vi "Config_PXDAC4800_2.vi"(0 "NumBoard":u32=1, 5 "Config":T2={"Clock source"=enum."1200 MHz", "Active channel"=enum."Dual channel - Ch1 & Ch2", "Trigger direction"=enum."Positive (Rising edge)", "Trigger mode"=enum."Continuous", "External Trigger enable"=FALSE, "Dac sample size"=enum."14 Bits LSB\n", "Dac sample format"=enum."Unsigned", "ClkDiv1"=1, "ClkDiv2"=1, "Output voltage level - Ch1"=1023, "Output voltage level - Ch2"=1023, "Output voltage level - Ch3"=1023, "Output voltage level - Ch4"=1023} {"Output voltage level - Ch4" min=1 max=1023 step=1 scale=0.0..1023.0; "Output voltage level - Ch3" min=1 max=1023 step=1 scale=0.0..1023.0; "Output voltage level - Ch2" min=1 max=1023 step=1 scale=0.0..1023.0; "Output voltage level - Ch1" min=1 max=1023 step=1 scale=0.0..1023.0}) -> (6 "Handle":u32=215368648, 8 "Serial num":u32=301738, 10 "Status":i32, 15 "Error/output message":string="SUCCESS")   [LabVIEW 2016]
panel:
  out "x+y":dbl=1.9797466172610085
  out "x*y":dbl=0.35000000000000003
  in  "NumBoard 3":u32=1
  in  "NumBoard 2":u32=1
  out "Serial num 3":u32=301738
  out "Handle 4":u32=266145720
  out "Status 4":i32
  out "Error/output message 4":string="SUCCESS"
  in  "Create Waveform":bool=TRUE
  in  "Playback":bool=TRUE
  in  "Configure":bool
  in  "Tab Control":T1(tab)=enum."Create Waveform"
  in  "DAC frequency (MHz)":dbl=1200.0
  in  "Number Of Points(integer multiple of 4096)":i32=30
  in  "Envelope Decay Time (micro s)":dbl=0.1
  in  "Amplitude (Max 1.4 V)":dbl=1.3
  in  "Frequency (MHz)":dbl=220.0
  out "output waveform":waveform(dbl)(graph)={"t0"=timestamp(0 s since 1904-01-01), "dt"=0.0008333333333333334, "Y"=array[122880 elements]}
  out "output waveform 2":waveform(dbl)(graph)={"t0"=timestamp(0 s since 1904-01-01), "dt"=0.0008333333333333334, "Y"=array[122880 elements]}
  in  "Shaped Wave Packet":bool=TRUE
  in  "Duty Cycle":dbl=2.0
  in  "Pulse Center":dbl=4.0
  in  "Square Pulse Amplitude":dbl=1.4 format="%#_13g"
  in  "Pulsed":bool=TRUE
  in  "VISA Refnum in":refnum<visa-resource-name>="USB0::0x0699::0x0353::1650390::INSTR"
  in  "time(us) 2":dbl=1.0
  out "Status 2":i32
  out "Handle 2":u32=266146304
  out "Serial num 2":u32=301738
  in  "dst_offset_bytes":u32
  in  "dst_length_bytes":u32
  in  "src_offset_bytes":u32
  in  "src_length_bytes":u32
  in  "Offset":u32
  in  "Length":u32
  out "Error/output message 3":string="SUCCESS"
  out "Channel":i32=3
  out "Handle 3":u32=264143912
  out "Status 3":i32
  in  "Run":bool=TRUE
  out "Error/output message 2":string="SUCCESS"
  in  "File":path=path "C:/Program Files (x86)/Signatec/PXDAC4800/version5.rd16"
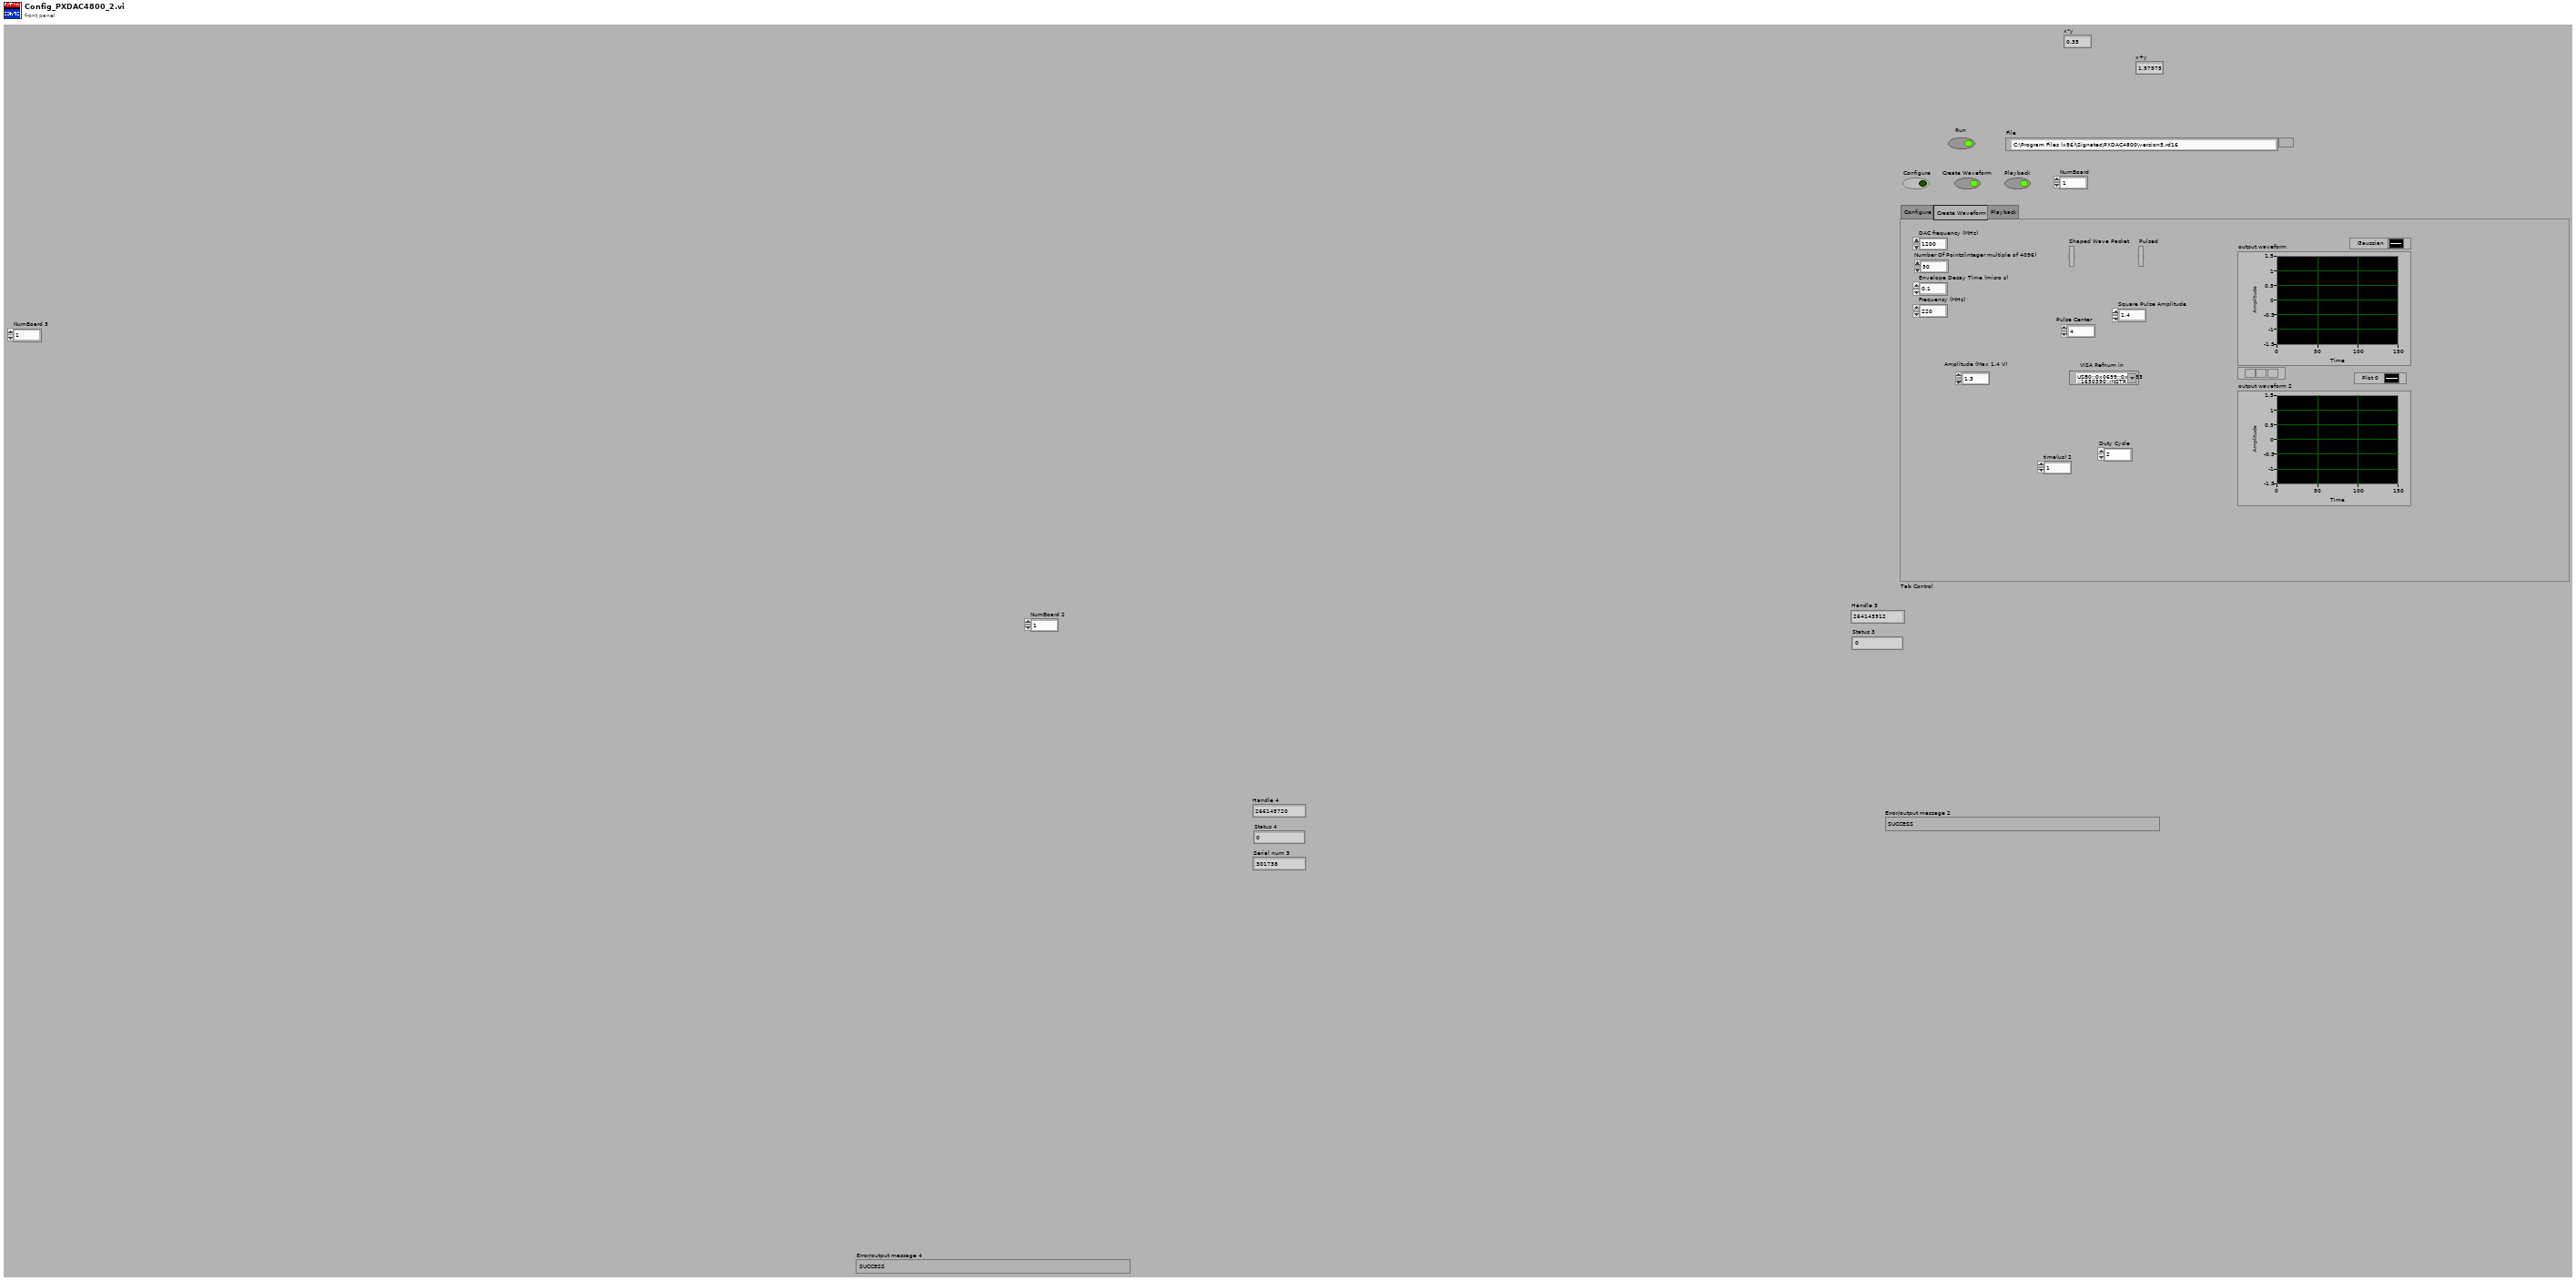
[diagram p1: front panel]
types:
  T1 = enum32{"Configure", "Create Waveform", "Playback"}
  T2 = cluster{"Clock source":enum16{"1200 MHz", "900 MHz", "External"}, "Active channel":enum16{"Dual channel - Ch1 & Ch2", "Single channel - Ch1"}, "Trigger direction":enum16{"Positive (Rising edge)", "Negative (Falling edge)"}, "Trigger mode":enum16{"Per trigger", "Continuous", "Single shot"}, "External Trigger enable":bool, "Dac sample size":enum16{"8 bits", "14 bits MSB", "14 Bits LSB\n"}, "Dac sample format":enum16{"Unsigned", "Signed"}, "ClkDiv1":u32, "ClkDiv2":u32, "Output voltage level - Ch1":u32, "Output voltage level - Ch2":u32, "Output voltage level - Ch3":u32, "Output voltage level - Ch4":u32}
  T3 = enum16{"Connect", "EndRamPlaybackXD48", "Disconnect"}
  T4 = enum16{"Connect", "GetSerialNumber", "SetActiveChannelMaskXD48", "SetPlaybackClockSourceXD48", "SetClockDivider1XD48", "SetClockDivider2XD48", "SetOutputVoltageCh1XD48", "SetOutputVoltageCh2XD48", "SetOutputVoltageCh3XD48", "SetOutputVoltageCh4XD48", "SetDacSampleFormatXD48", "SetDacSampleSizeXD48", "SetExternalTriggerEnableXD48", "SetExternalTriggerDirXD48", "SetTriggerModeXD48", "Disconnect"}
  T5 = enum16{"Dual channel - Ch1 & Ch2", "Single channel - Ch1"}
  T6 = enum16{"Positive (Rising edge)", "Negative (Falling edge)"}
  T7 = enum16{"Per trigger", "Continuous", "Single shot"}
  T8 = enum16{"Connect", "GetSerialNumber", "EndRamPlaybackXD48"}
  T9 = enum16{"Connect", "GetSerialNumber", "LoadFileIntoRam", "BeginRamPlayback", "Trigger", "EndRamPlaybackXD48", "Disconnect"}
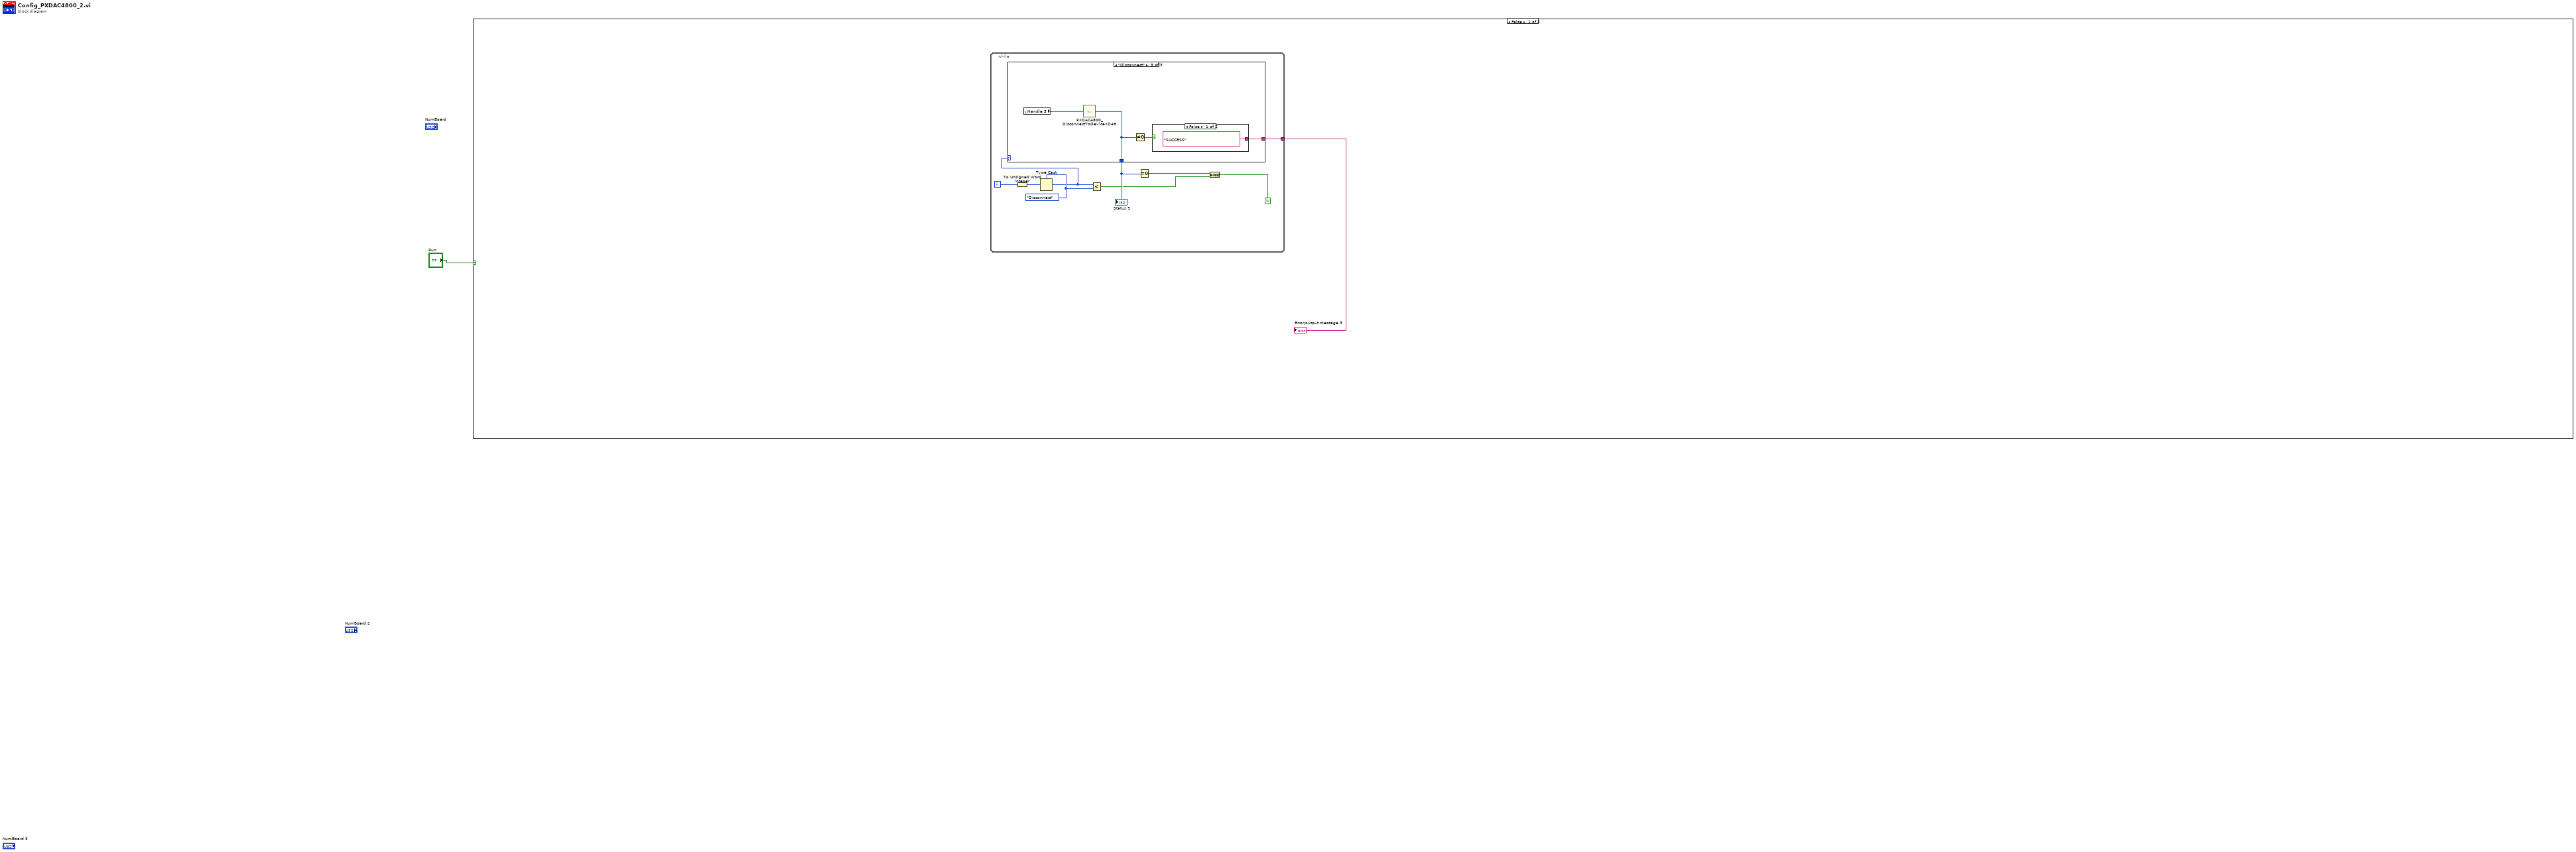
[diagram p0: block diagram]
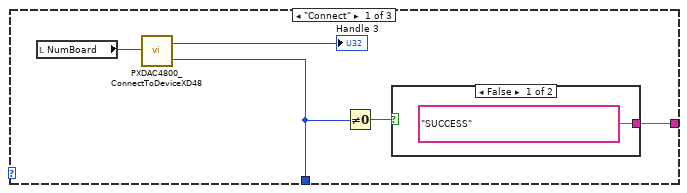
[diagram p2: hidden frame]
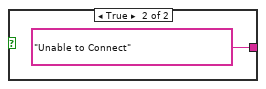
[diagram p3: hidden frame]
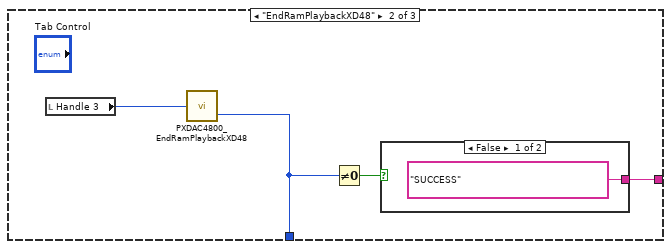
[diagram p4: hidden frame]
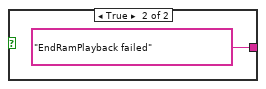
[diagram p5: hidden frame]
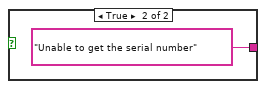
[diagram p6: hidden frame]
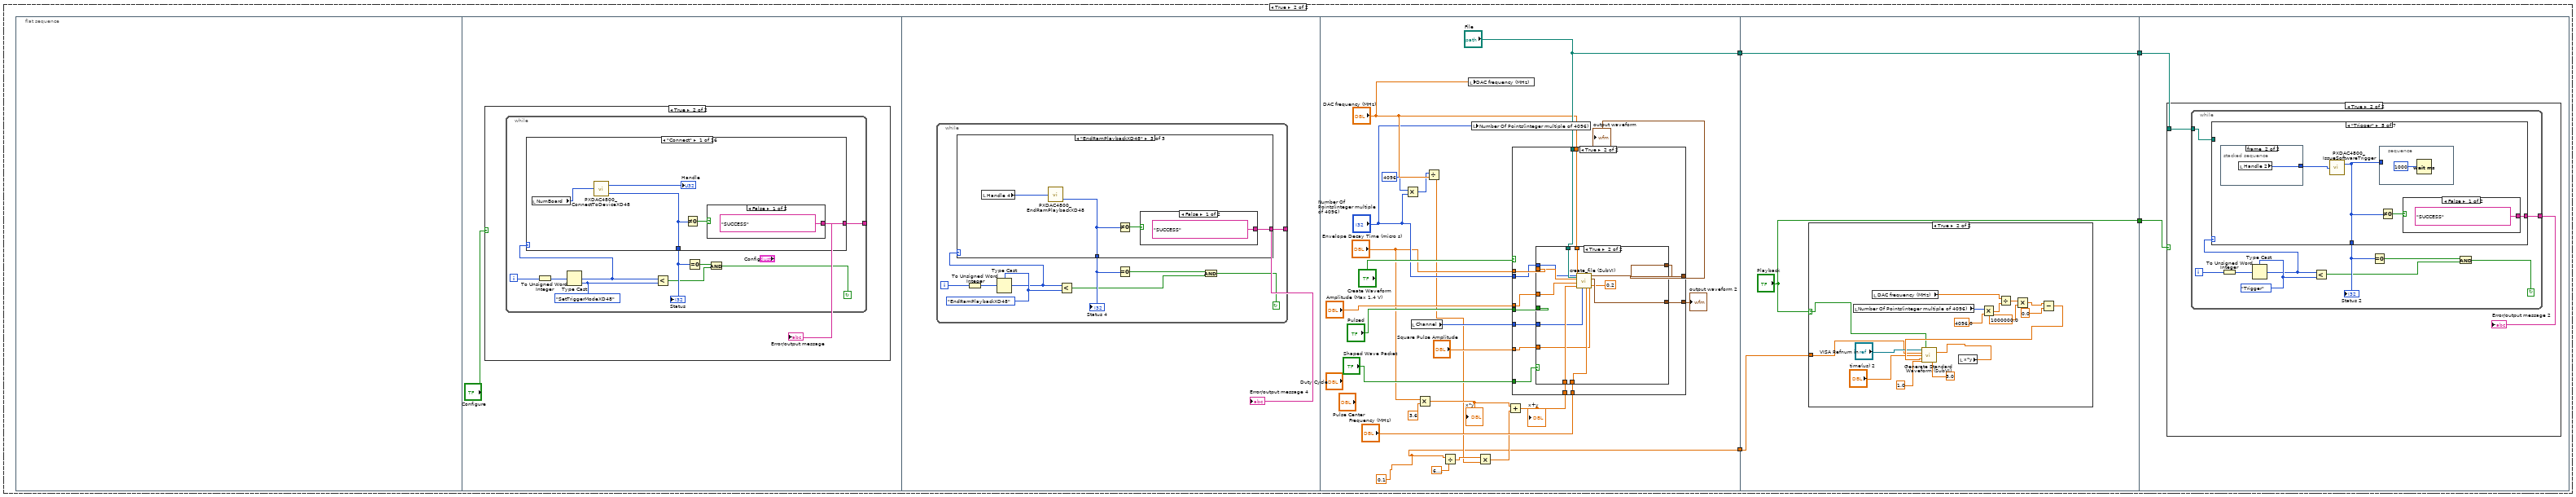
[diagram p7: hidden frame]
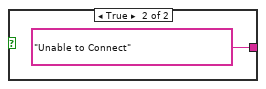
[diagram p9: hidden frame]
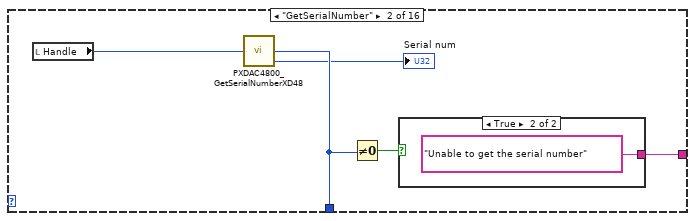
[diagram p10: hidden frame]
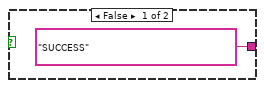
[diagram p11: hidden frame]
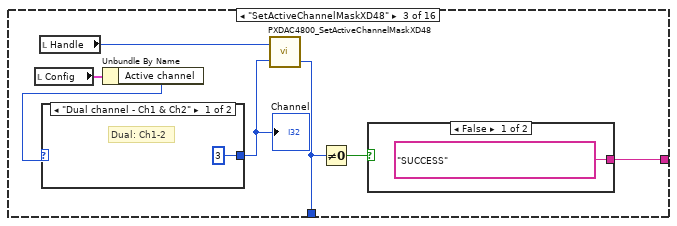
[diagram p12: hidden frame]
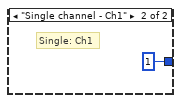
[diagram p13: hidden frame]
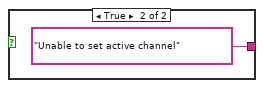
[diagram p14: hidden frame]
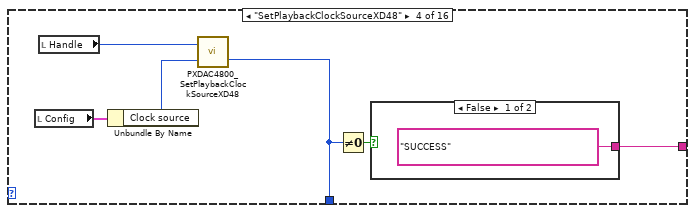
[diagram p15: hidden frame]
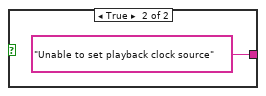
[diagram p16: hidden frame]
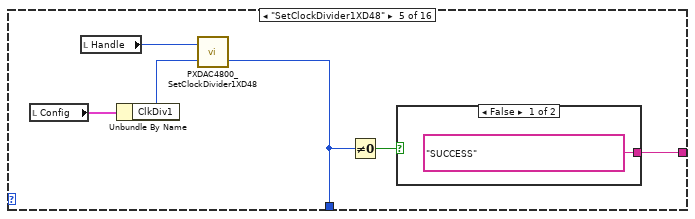
[diagram p17: hidden frame]
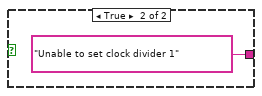
[diagram p18: hidden frame]
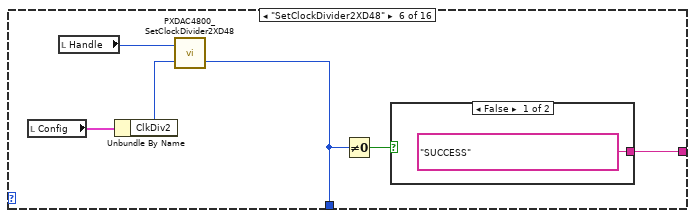
[diagram p19: hidden frame]
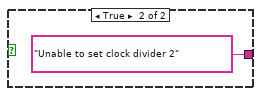
[diagram p20: hidden frame]
diagram:
  n1 = case shown="False" "Run" {
    frame False {
      n2 = while {
        tunnel: [w4] -> w2
        i -> [w11]
        stop <- w5 continue-if-true
        w9 = T3."Disconnect"
        n3 = To Unsigned Word Integer(number=w11) -> (unsigned 16bit integer=w10:u16)
        n4 = Type Cast(type=w9, x=w10) -> (*(type *) &x=w3:T3)
        n5 = case shown="\"Disconnect\"" w3 {
          tunnel: [w13 w19 w25] -> w8
          tunnel: [w15 w21 w28] -> w4
          frame "Connect" {
            n6 = local read "NumBoard"() -> (w12:u32)
            n7 = call "PXDAC4800_ConnectToDeviceXD48.vi"("brdNum"=w12) -> ("Handle Out"=→"Handle 3":i32, "Status"=w13:i32)
            n8 = Not Equal To 0?(x=w13) -> (x != 0?=w16:bool)
            n9 = case shown="False" w16 {
              tunnel: ["SUCCESS" "Unable to Connect"] -> w15
              frame False {
              }
              frame True {
              }
            }
          }
          frame "EndRamPlaybackXD48" {
            n10 = local read "Handle 3"() -> (w20:u32)
            n11 = call "PXDAC4800_EndRamPlaybackXD48.vi"("Handle"=w20) -> ("Status"=w19:i32)  [unwired: 1 out]
            n12 = Not Equal To 0?(x=w19) -> (x != 0?=w22:bool)
            n13 = case shown="False" w22 {
              tunnel: ["SUCCESS" "EndRamPlayback failed"] -> w21
              frame False {
              }
              frame True {
              }
            }
          }
          frame "Disconnect" {
            n14 = local read "Handle 3"() -> (w26:u32)
            n15 = call "PXDAC4800_DisconnectToDeviceXD48.vi"("Handle"=w26) -> ("Status"=w25:i32)
            n16 = Not Equal To 0?(x=w25) -> (x != 0?=w27:bool)
            n17 = case shown="False" w27 {
              tunnel: ["SUCCESS" "Unable to get the serial number"] -> w28
              frame False {
              }
              frame True {
              }
            }
          }
        }
        "Status 3" <- w8
        n18 = Less?(x=w3, y=w9) -> (x < y?=w6:bool)
        n19 = Equal To 0?(x=w8) -> (x = 0?=w7:bool)
        n20 = And(x=w7, y=w6) -> (x .and. y?=w5:bool)
      }
      "Error/output message 3" <- w2
    }
    frame True {
      n21 = flat-sequence {
        tunnel: ["File"] -> w34
        tunnel: [w206] -> w31
        tunnel: w34 -> [w293]
        tunnel: [w293] -> w33
        tunnel: ["Playback"] -> w32
        tunnel: w31 -> [w291]
        tunnel: w33 -> [w311]
        tunnel: w32 -> [w310]
        frame #0 {
        }
        frame #1 {
          n22 = case shown="True" "Configure" {
            frame False {
            }
            frame True {
              n23 = while {
                tunnel: [w37] -> w36
                i -> [w45]
                stop <- w38 continue-if-true
                w42 = T4."SetTriggerModeXD48"
                n24 = To Unsigned Word Integer(number=w45) -> (unsigned 16bit integer=w44:u16)
                n25 = Type Cast(type=w42, x=w44) -> (*(type *) &x=w43:T4)
                n26 = case shown="\"Connect\"" w43 {
                  tunnel: [w47 w55 w64 w74 w81 w89 w97 w105 w113 w121 w129 w137 w145 w156 w164 w170] -> w41
                  tunnel: [w49 w56 w65 w75 w83 w91 w99 w107 w115 w123 w131 w139 w148 w158 w166 w173] -> w37
                  frame "Connect" {
                    n27 = local read "NumBoard"() -> (w46:u32)
                    n28 = call "PXDAC4800_ConnectToDeviceXD48.vi"("brdNum"=w46) -> ("Handle Out"=→"Handle":i32, "Status"=w47:i32)
                    n29 = Not Equal To 0?(x=w47) -> (x != 0?=w50:bool)
                    n30 = case shown="False" w50 {
                      tunnel: ["SUCCESS" "Unable to Connect"] -> w49
                      frame False {
                      }
                      frame True {
                      }
                    }
                  }
                  frame "GetSerialNumber" {
                    (unwired) "Unable to get serial"
                    n31 = local read "Handle"() -> (w53:u32)
                    n32 = call "PXDAC4800_GetSerialNumberXD48.vi"("Handle"=w53) -> ("Status"=w55:i32, "Serial num"=→"Serial num":i32)  [unwired: 1 out]
                    n33 = Not Equal To 0?(x=w55) -> (x != 0?=w57:bool)
                    n34 = case shown="True" w57 {
                      tunnel: ["SUCCESS" "Unable to get the serial number"] -> w56
                      frame False {
                      }
                      frame True {
                      }
                    }
                  }
                  frame "SetActiveChannelMaskXD48" {
                    n35 = local read "Config"() -> (w63:T2)
                    n36 = local read "Handle"() -> (w61:u32)
                    n37 = Unbundle By Name(w63) -> ("Active channel"=w62:T5)
                    n38 = case shown="\"Dual channel - Ch1 & Ch2\"" w62 {
                      tunnel: [3 1] -> w60
                      frame "Dual channel - Ch1 & Ch2" {
                        # "Dual: Ch1-2"
                      }
                      frame "Single channel - Ch1" {
                        # "Single: Ch1"
                      }
                    }
                    "Channel" <- w60
                    n39 = call "PXDAC4800_SetActiveChannelMaskXD48.vi"("Value"=w60, "Handle"=w61) -> ("Status"=w64:i32)  [unwired: 1 out]
                    n40 = Not Equal To 0?(x=w64) -> (x != 0?=w66:bool)
                    n41 = case shown="False" w66 {
                      tunnel: ["SUCCESS" "Unable to set active channel"] -> w65
                      frame False {
                      }
                      frame True {
                      }
                    }
                  }
                  frame "SetPlaybackClockSourceXD48" {
                    n42 = local read "Config"() -> (w72:T2)
                    n43 = local read "Handle"() -> (w73:u32)
                    n44 = Unbundle By Name(w72) -> ("Clock source"=w71:enum16{"1200 MHz", "900 MHz", "External"})
                    n45 = call "PXDAC4800_SetPlaybackClockSourceXD48.vi"("Value"=w71, "Handle"=w73) -> ("Status"=w74:i32)  [unwired: 1 out]
                    n46 = Not Equal To 0?(x=w74) -> (x != 0?=w76:bool)
                    n47 = case shown="False" w76 {
                      tunnel: ["SUCCESS" "Unable to set playback clock source"] -> w75
                      frame False {
                      }
                      frame True {
                      }
                    }
                  }
                  frame "SetClockDivider1XD48" {
                    n48 = local read "Config"() -> (w80:T2)
                    n49 = local read "Handle"() -> (w82:u32)
                    n50 = Unbundle By Name(w80) -> ("ClkDiv1"=w79:u32)
                    n51 = call "PXDAC4800_SetClockDivider1XD48.vi"("Div"=w79, "Handle"=w82) -> ("Status"=w81:i32)  [unwired: 1 out]
                    n52 = Not Equal To 0?(x=w81) -> (x != 0?=w84:bool)
                    n53 = case shown="False" w84 {
                      tunnel: ["SUCCESS" "Unable to set clock divider 1"] -> w83
                      frame False {
                      }
                      frame True {
                      }
                    }
                  }
                  frame "SetClockDivider2XD48" {
                    n54 = local read "Config"() -> (w88:T2)
                    n55 = local read "Handle"() -> (w90:u32)
                    n56 = Unbundle By Name(w88) -> ("ClkDiv2"=w87:u32)
                    n57 = call "PXDAC4800_SetClockDivider2XD48.vi"("Div"=w87, "Handle"=w90) -> ("Status"=w89:i32)  [unwired: 1 out]
                    n58 = Not Equal To 0?(x=w89) -> (x != 0?=w92:bool)
                    n59 = case shown="False" w92 {
                      tunnel: ["SUCCESS" "Unable to set clock divider 2"] -> w91
                      frame False {
                      }
                      frame True {
                      }
                    }
                  }
                  frame "SetOutputVoltageCh1XD48" {
                    n60 = local read "Config"() -> (w96:T2)
                    n61 = local read "Handle"() -> (w98:u32)
                    n62 = Unbundle By Name(w96) -> ("Output voltage level - Ch1"=w95:u32)
                    n63 = call "PXDAC4800_SetOutputVoltageCh1XD48.vi"("Value"=w95, "Handle"=w98) -> ("Status"=w97:i32)  [unwired: 1 out]
                    n64 = Not Equal To 0?(x=w97) -> (x != 0?=w100:bool)
                    n65 = case shown="False" w100 {
                      tunnel: ["SUCCESS" "Unable to set output voltage range ch1"] -> w99
                      frame False {
                      }
                      frame True {
                      }
                    }
                  }
                  frame "SetOutputVoltageCh2XD48" {
                    n66 = local read "Config"() -> (w104:T2)
                    n67 = local read "Handle"() -> (w106:u32)
                    n68 = Unbundle By Name(w104) -> ("Output voltage level - Ch2"=w103:u32)
                    n69 = call "PXDAC4800_SetOutputVoltageCh2XD48.vi"("Value"=w103, "Handle"=w106) -> ("Status"=w105:i32)  [unwired: 1 out]
                    n70 = Not Equal To 0?(x=w105) -> (x != 0?=w108:bool)
                    n71 = case shown="False" w108 {
                      tunnel: ["SUCCESS" "Unable to set output voltage range ch2"] -> w107
                      frame False {
                      }
                      frame True {
                      }
                    }
                  }
                  frame "SetOutputVoltageCh3XD48" {
                    n72 = local read "Config"() -> (w112:T2)
                    n73 = local read "Handle"() -> (w114:u32)
                    n74 = Unbundle By Name(w112) -> ("Output voltage level - Ch3"=w111:u32)
                    n75 = call "PXDAC4800_SetOutputVoltageCh3XD48.vi"("Value"=w111, "Handle"=w114) -> ("Status"=w113:i32)  [unwired: 1 out]
                    n76 = Not Equal To 0?(x=w113) -> (x != 0?=w116:bool)
                    n77 = case shown="False" w116 {
                      tunnel: ["SUCCESS" "Unable to set output voltage range ch3"] -> w115
                      frame False {
                      }
                      frame True {
                      }
                    }
                  }
                  frame "SetOutputVoltageCh4XD48" {
                    n78 = local read "Config"() -> (w120:T2)
                    n79 = local read "Handle"() -> (w122:u32)
                    n80 = Unbundle By Name(w120) -> ("Output voltage level - Ch4"=w119:u32)
                    n81 = call "PXDAC4800_SetOutputVoltageCh4XD48.vi"("Value"=w119, "Handle"=w122) -> ("Status"=w121:i32)  [unwired: 1 out]
                    n82 = Not Equal To 0?(x=w121) -> (x != 0?=w124:bool)
                    n83 = case shown="False" w124 {
                      tunnel: ["SUCCESS" "Unable to set output voltage range ch4"] -> w123
                      frame False {
                      }
                      frame True {
                      }
                    }
                  }
                  frame "SetDacSampleFormatXD48" {
                    n84 = local read "Config"() -> (w128:T2)
                    n85 = local read "Handle"() -> (w130:u32)
                    n86 = Unbundle By Name(w128) -> ("Dac sample format"=w127:enum16{"Unsigned", "Signed"})
                    n87 = call "PXDAC4800_SetDacSampleFormatXD48.vi"("Value"=w127, "Handle"=w130) -> ("Status"=w129:i32)  [unwired: 1 out]
                    n88 = Not Equal To 0?(x=w129) -> (x != 0?=w132:bool)
                    n89 = case shown="False" w132 {
                      tunnel: ["SUCCESS" "Unable to set Dac sample format"] -> w131
                      frame False {
                      }
                      frame True {
                      }
                    }
                  }
                  frame "SetDacSampleSizeXD48" {
                    n90 = local read "Config"() -> (w136:T2)
                    n91 = local read "Handle"() -> (w138:u32)
                    n92 = Unbundle By Name(w136) -> ("Dac sample size"=w135:enum16{"8 bits", "14 bits MSB", "14 Bits LSB\n"})
                    n93 = call "PXDAC4800_SetDacSampleSizeXD48.vi"("Value"=w135, "Handle"=w138) -> ("Status"=w137:i32)  [unwired: 1 out]
                    n94 = Not Equal To 0?(x=w137) -> (x != 0?=w140:bool)
                    n95 = case shown="False" w140 {
                      tunnel: ["SUCCESS" "Unable to set sample size"] -> w139
                      frame False {
                      }
                      frame True {
                      }
                    }
                  }
                  frame "SetExternalTriggerEnableXD48" {
                    n96 = local read "Config"() -> (w144:T2)
                    n97 = local read "Handle"() -> (w147:u32)
                    n98 = Unbundle By Name(w144) -> ("External Trigger enable"=w143:bool)
                    n99 = case shown="False" w143 {
                      tunnel: [0 1] -> w146
                      frame False {
                      }
                      frame True {
                      }
                    }
                    n100 = call "PXDAC4800_SetExternalTriggerEnableXD48.vi"("bEnable"=w146, "Handle"=w147) -> ("Status"=w145:i32)  [unwired: 1 out]
                    n101 = Not Equal To 0?(x=w145) -> (x != 0?=w149:bool)
                    n102 = case shown="False" w149 {
                      tunnel: ["SUCCESS" "Unable to set external trigger enable"] -> w148
                      frame False {
                      }
                      frame True {
                      }
                    }
                  }
                  frame "SetExternalTriggerDirXD48" {
                    n103 = local read "Config"() -> (w155:T2)
                    n104 = local read "Handle"() -> (w157:u32)
                    n105 = Unbundle By Name(w155) -> ("Trigger direction"=w154:T6)
                    n106 = call "PXDAC4800_SetExternalTriggerDirXD48.vi"("Value"=w154, "Handle"=w157) -> ("Status"=w156:i32)  [unwired: 1 out]
                    n107 = Not Equal To 0?(x=w156) -> (x != 0?=w159:bool)
                    n108 = case shown="False" w159 {
                      tunnel: ["SUCCESS" "Unable to set external trigger direction"] -> w158
                      frame False {
                      }
                      frame True {
                      }
                    }
                  }
                  frame "SetTriggerModeXD48" {
                    n109 = local read "Config"() -> (w163:T2)
                    n110 = local read "Handle"() -> (w165:u32)
                    n111 = Unbundle By Name(w163) -> ("Trigger mode"=w162:T7)
                    n112 = call "PXDAC4800_SetTriggerModeXD48.vi"("Value"=w162, "Handle"=w165) -> ("Status"=w164:i32)  [unwired: 1 out]
                    n113 = Not Equal To 0?(x=w164) -> (x != 0?=w167:bool)
                    n114 = case shown="False" w167 {
                      tunnel: ["SUCCESS" "Unable to set trigger mode"] -> w166
                      frame False {
                      }
                      frame True {
                      }
                    }
                  }
                  frame "Disconnect" {
                    n115 = local read "Handle"() -> (w171:u32)
                    n116 = call "PXDAC4800_DisconnectToDeviceXD48.vi"("Handle"=w171) -> ("Status"=w170:i32)
                    n117 = Not Equal To 0?(x=w170) -> (x != 0?=w172:bool)
                    n118 = case shown="False" w172 {
                      tunnel: ["SUCCESS" "Unable to disconnect"] -> w173
                      frame False {
                      }
                      frame True {
                      }
                    }
                  }
                }
                "Status" <- w41
                n119 = Less?(x=w43, y=w42) -> (x < y?=w39:bool)
                n120 = Equal To 0?(x=w41) -> (x = 0?=w40:bool)
                n121 = And(x=w40, y=w39) -> (x .and. y?=w38:bool)
              }
              "Error/output message" <- w36
            }
          }
        }
        frame #2 {
          n122 = while {
            tunnel: [w178] -> w176
            i -> [w185]
            stop <- w179 continue-if-true
            w183 = T8."EndRamPlaybackXD48"
            n123 = To Unsigned Word Integer(number=w185) -> (unsigned 16bit integer=w184:u16)
            n124 = Type Cast(type=w183, x=w184) -> (*(type *) &x=w177:T8)
            n125 = case shown="\"EndRamPlaybackXD48\"" w177 {
              tunnel: [w187 w193 w200] -> w182
              tunnel: [w189 w196 w202] -> w178
              frame "Connect" {
                n126 = local read "NumBoard 2"() -> (w186:u32)
                n127 = call "PXDAC4800_ConnectToDeviceXD48.vi"("brdNum"=w186) -> ("Handle Out"=→"Handle 4":i32, "Status"=w187:i32)
                n128 = Not Equal To 0?(x=w187) -> (x != 0?=w190:bool)
                n129 = case shown="False" w190 {
                  tunnel: ["SUCCESS" "Unable to Connect"] -> w189
                  frame False {
                  }
                  frame True {
                  }
                }
              }
              frame "GetSerialNumber" {
                (unwired) "Unable to get serial"
                n130 = local read "Handle 4"() -> (w195:u32)
                n131 = call "PXDAC4800_GetSerialNumberXD48.vi"("Handle"=w195) -> ("Status"=w193:i32, "Serial num"=→"Serial num 3":i32)  [unwired: 1 out]
                n132 = Not Equal To 0?(x=w193) -> (x != 0?=w197:bool)
                n133 = case shown="False" w197 {
                  tunnel: ["SUCCESS" "Unable to get the serial number"] -> w196
                  frame False {
                  }
                  frame True {
                  }
                }
              }
              frame "EndRamPlaybackXD48" {
                n134 = local read "Handle 4"() -> (w201:u32)
                n135 = call "PXDAC4800_EndRamPlaybackXD48.vi"("Handle"=w201) -> ("Status"=w200:i32)  [unwired: 1 out]
                n136 = Not Equal To 0?(x=w200) -> (x != 0?=w203:bool)
                n137 = case shown="False" w203 {
                  tunnel: ["SUCCESS" "EndRamPlayback failed"] -> w202
                  frame False {
                  }
                  frame True {
                  }
                }
              }
            }
            "Status 4" <- w182
            n138 = Less?(x=w177, y=w183) -> (x < y?=w180:bool)
            n139 = Equal To 0?(x=w182) -> (x = 0?=w181:bool)
            n140 = And(x=w181, y=w180) -> (x .and. y?=w179:bool)
          }
          "Error/output message 4" <- w176
        }
        frame #3 {
          w206 = 0.1 ("y")
          n141 = Multiply(x=4096, y="Number Of Points(integer multiple of 4096)") -> (x*y=w216:i32)
          n142 = local read "Channel"() -> (w223:i32)
          n143 = Multiply(x="Envelope Decay Time (micro s)", y=3.6) -> (x*y=w210:dbl)
          "x*y" <- w210
          n144 = Divide(x=w216, y="DAC frequency (MHz)") -> (x/y=w207:dbl)
          n145 = Divide(x=w206, y=6.283185307179586) -> (x/y=w211:dbl)
          n146 = local write "DAC frequency (MHz)"("DAC frequency (MHz)") -> ()
          n147 = local write "Number Of Points(integer multiple of 4096)"("Number Of Points(integer multiple of 4096)") -> ()
          n148 = Multiply(x=w211, y=w207) -> (x*y=w209:dbl)
          n149 = Add(x=w210, y=w209) -> (x+y=w208:dbl)
          "x+y" <- w208
          n150 = case shown="True" "Create Waveform" {
            tunnel: "File" -> [_ w240]
            tunnel: "DAC frequency (MHz)" -> [_ w239]
            tunnel: "Number Of Points(integer multiple of 4096)" -> [_ w236]
            tunnel: "Envelope Decay Time (micro s)" -> [_ w237]
            tunnel: "Amplitude (Max 1.4 V)" -> [_ w238]
            tunnel: "Frequency (MHz)" -> [_ w242]
            tunnel: [w230 w235] -> w226
            tunnel: w208 -> [_ w243]
            tunnel: "Shaped Wave Packet" -> [_ w241]
            tunnel: w223 -> [_ w234]
            tunnel: "Square Pulse Amplitude" -> [_ w233]
            tunnel: [w229 w232] -> w221
            tunnel: "Pulsed" -> [_ w231]
            frame False {
              n151 = local read "output waveform 2"() -> (w229:waveform(dbl))
              n152 = local read "output waveform"() -> (w230:waveform(dbl))
            }
            frame True {
              n153 = case shown="True" w241 {
                tunnel: w242 -> [w248 w283]
                tunnel: [w255 w290] -> w235
                tunnel: w236 -> [w250 w284]
                tunnel: w240 -> [w251 w289]
                tunnel: w239 -> [w252 w288]
                tunnel: w237 -> [w254 w287]
                tunnel: w238 -> [w253 w286]
                tunnel: w243 -> [w249 w285]
                tunnel: w234 -> [w245 w282]
                tunnel: w233 -> [w246 w281]
                tunnel: [w247 w280] -> w232
                tunnel: w231 -> [w244 _]
                frame False {
                  n154 = case shown="True" w244 {
                    tunnel: [w264 w278] -> w255
                    tunnel: w254 -> [w257 w277]
                    tunnel: w253 -> [w256 w275]
                    tunnel: w252 -> [w261 w273]
                    tunnel: w251 -> [w260 w272]
                    tunnel: w250 -> [_ w271]
                    tunnel: w249 -> [_ w270]
                    tunnel: w248 -> [w259 w269]
                    tunnel: [w263 w268] -> w247
                    tunnel: w246 -> [w258 w267]
                    tunnel: w245 -> [w262 w266]
                    frame False {
                      n155 = call "continuous_sin.vi"("file path (use dialog)"=w260, "Amplitude"=w256, "Frequency (MHz)"=w259, "Numeric"=w262, "Trigger Width (us)"=w257, "Pulse Amplitude"=w258, "DAC frequency (MHz)"=w261) -> ("output waveform 2"=w263:waveform(dbl), "output waveform"=w264:waveform(dbl))  [unwired: 3 in]
                    }
                    frame True {
                      n156 = Multiply(x=w277, y=6.0) -> (x*y=w274:dbl)
                      n157 = call "create_file_sin (SubVI).vi"("Channel"=w266, "Trigger Width"=0.1, "Frequency (MHz)"=w269, "Square Pulse Amplitude"=w267, "Amplitude"=w275, "Pulse Width"=w274, "Number Of Points(integer multiple of 4096)"=w271, "DAC frequency (MHz)"=w273, "Pulse Center"=w270, "file path (use dialog)"=w272) -> ("output waveform 2"=w268:waveform(dbl), "output waveform"=w278:waveform(dbl))
                    }
                  }
                }
                frame True {
                  n158 = call "create_file (SubVI).vi"("Pulse Amplitude"=w281, "Trigger Width (us)"=0.2, "Frequency (MHz)"=w283, "DAC frequency (MHz)"=w288, "Numeric"=w282, "file path (use dialog)"=w289, "Pulse Center"=w285, "Amplitude"=w286, "Envelope Decay Time (micro s)"=w287, "Number Of Points(integer multiple of 4096)"=w284) -> ("output waveform 2"=w280:waveform(dbl), "output waveform"=w290:waveform(dbl))
                }
              }
            }
          }
          "output waveform" <- w226
          "output waveform 2" <- w221
        }
        frame #4 {
          n159 = case shown="True" "Playback" {
            selector: "Playback" -> [_ w295]
            tunnel: w291 -> [_ w294]
            frame False {
            }
            frame True {
              n160 = local read "Number Of Points(integer multiple of 4096)"() -> (w296:i32)
              n161 = local read "DAC frequency (MHz)"() -> (w299:dbl)
              n162 = local read "x*y"() -> (w309:dbl)
              n163 = Multiply(x=w296, y=4096.0) -> (x*y=w298:dbl)
              n164 = Divide(x=w299, y=w298) -> (x/y=w300:dbl)
              n165 = Multiply(x=w300, y=1000000.0) -> (x*y=w306:dbl)
              n166 = Subtract(x=w306, y=0.0) -> (x-y=w308:dbl)
              n167 = call "Generate Standard Waveform (SubVI).vi"("VISA Refnum in"="VISA Refnum in", "Enable Output (T: Enable)"=w295, "Envelope Decay Time"=w309, "Phase Before Trigger"=w294, "time (us)"="time(us) 2", "Frequency (1000 Hz)"=w308, "t before"=1.0, "Amplitude (1 Vpp)"=3.0) -> ()  [unwired: 8 in]
            }
          }
        }
        frame #5 {
          n168 = case shown="True" w310 {
            tunnel: w311 -> [_ w312]
            frame False {
            }
            frame True {
              n169 = while {
                tunnel: [w316] -> w313
                tunnel: w312 -> [w314]
                i -> [w323]
                stop <- w317 continue-if-true
                w321 = T9."Trigger"
                n170 = To Unsigned Word Integer(number=w323) -> (unsigned 16bit integer=w322:u16)
                n171 = Type Cast(type=w321, x=w322) -> (*(type *) &x=w315:T9)
                n172 = case shown="\"Trigger\"" w315 {
                  tunnel: [w325 w331 w341 w360 w368 w376 w382] -> w320
                  tunnel: [w327 w334 w347 w362 w369 w378 w385] -> w316
                  tunnel: w314 -> [_ _ w338 _ _ _ _]
                  frame "Connect" {
                    n173 = local read "NumBoard"() -> (w324:u32)
                    n174 = call "PXDAC4800_ConnectToDeviceXD48.vi"("brdNum"=w324) -> ("Handle Out"=→"Handle 2":i32, "Status"=w325:i32)
                    n175 = Not Equal To 0?(x=w325) -> (x != 0?=w328:bool)
                    n176 = case shown="False" w328 {
                      tunnel: ["SUCCESS" "Unable to Connect"] -> w327
                      frame False {
                      }
                      frame True {
                      }
                    }
                  }
                  frame "GetSerialNumber" {
                    (unwired) "Unable to get serial"
                    n177 = local read "Handle 2"() -> (w333:u32)
                    n178 = call "PXDAC4800_GetSerialNumberXD48.vi"("Handle"=w333) -> ("Status"=w331:i32, "Serial num"=→"Serial num 2":i32)  [unwired: 1 out]
                    n179 = Not Equal To 0?(x=w331) -> (x != 0?=w335:bool)
                    n180 = case shown="False" w335 {
                      tunnel: ["SUCCESS" "Unable to get the serial number"] -> w334
                      frame False {
                      }
                      frame True {
                      }
                    }
                  }
                  frame "LoadFileIntoRam" {
                    n181 = Path To String(path=w338) -> (string=w339:string)
                    n182 = local read "Handle 2"() -> (w340:u32)
                    n183 = call "PXDAC4800_LoadFileIntoRamXD48.vi"("dst_offset_bytes"="dst_offset_bytes", "Handle"=w340, "dst_length_bytes"="dst_length_bytes", "src_offset_bytes"="src_offset_bytes", "src_length_bytes"="src_length_bytes", "File_Path"=w339) -> ("Status"=w341:i32)  [unwired: 1 in, 1 out]
                    n184 = Not Equal To 0?(x=w341) -> (x != 0?=w346:bool)
                    n185 = case shown="False" w346 {
                      tunnel: ["SUCCESS" "Unable to load the file into ram"] -> w347
                      frame False {
                      }
                      frame True {
                      }
                    }
                  }
                  frame "BeginRamPlayback" {
                    n186 = local read "Handle 2"() -> (w350:u32)
                    n187 = call "PXDAC4800_GetActiveMemoryRegionXD48.vi"("Handle"=w350, "Offset"="Offset", "Length Byte"="Length") -> ("Status"=w357:i32, "Handle out"=w356:u32, "Offset_bytes out"=w355:u32, "Playback_bytes out"=w354:u32)
                    n188 = call "PXDAC4800_BeginRamPlaybackXD48.vi"("ram length bytes"=w354, "ram offset bytes"=w355, "Handle"=w356) -> ("Status"=w351:i32)  [unwired: 1 in, 1 out]
                    n189 = Not Equal To 0?(x=w357) -> (x != 0?=w361:bool)
                    n190 = Not Equal To 0?(x=w351) -> (x != 0?=w359:bool)
                    n191 = Or(x=w361, y=w359) -> (x .or. y?=w358:bool)
                    n192 = case shown="False" w358 {
                      tunnel: ["SUCCESS" "Unable to begin the ram playback"] -> w362
                      tunnel: [0 -565] -> w360
                      frame False {
                      }
                      frame True {
                      }
                    }
                  }
                  frame "Trigger" {
                    n193 = stacked-sequence {
                      tunnel: [_ w373] -> w367
                      frame #0 {
                        n194 = Wait (ms)(milliseconds to wait=1000) -> ()  [unwired: 1 out]
                      }
                      frame #1 {
                        n195 = local read "Handle 2"() -> (w373:u32)
                      }
                    }
                    n196 = call "PXDAC4800_IssueSoftwareTrigger.vi"("Handle"=w367) -> ("Status"=w368:i32)  [unwired: 1 out]
                    n197 = stacked-sequence {
                      tunnel: w368 -> [_]
                      frame #0 {
                        n198 = Wait (ms)(milliseconds to wait=1000) -> ()  [unwired: 1 out]
                      }
                    }
                    n199 = Not Equal To 0?(x=w368) -> (x != 0?=w370:bool)
                    n200 = case shown="False" w370 {
                      tunnel: ["SUCCESS" "Trigger failed"] -> w369
                      frame False {
                      }
                      frame True {
                      }
                    }
                  }
                  frame "EndRamPlaybackXD48" {
                    n201 = local read "Handle 2"() -> (w377:u32)
                    n202 = call "PXDAC4800_EndRamPlaybackXD48.vi"("Handle"=w377) -> ("Status"=w376:i32)  [unwired: 1 out]
                    n203 = Not Equal To 0?(x=w376) -> (x != 0?=w379:bool)
                    n204 = case shown="False" w379 {
                      tunnel: ["SUCCESS" "EndRamPlayback failed"] -> w378
                      frame False {
                      }
                      frame True {
                      }
                    }
                  }
                  frame "Disconnect" {
                    n205 = local read "Handle 2"() -> (w383:u32)
                    n206 = call "PXDAC4800_DisconnectToDeviceXD48.vi"("Handle"=w383) -> ("Status"=w382:i32)
                    n207 = Not Equal To 0?(x=w382) -> (x != 0?=w384:bool)
                    n208 = case shown="False" w384 {
                      tunnel: ["SUCCESS" "Unable to get the serial number"] -> w385
                      frame False {
                      }
                      frame True {
                      }
                    }
                  }
                }
                "Status 2" <- w320
                n209 = Less?(x=w315, y=w321) -> (x < y?=w318:bool)
                n210 = Equal To 0?(x=w320) -> (x = 0?=w319:bool)
                n211 = And(x=w319, y=w318) -> (x .and. y?=w317:bool)
              }
              "Error/output message 2" <- w313
            }
          }
        }
      }
    }
  }
